vi "Configure Setpoints Limits.vi"(7 "Unit Address (1)":u8=1, 8 "error in (no error)":errorcluster, 9 "Setpoint Limit Value (0)":i16, 10 "Limit Type (False)":bool, 11 "VISA resource name":refnum<visa-resource-name>) -> (0 "error out":errorcluster, 3 "VISA resource name out":refnum<visa-resource-name>)   [LabVIEW 2014, in "Eurotherm 35xx Series.lvlib"]
doc: "This VI sets Setpoints limits."
uses:
  <instrlib>/Eurotherm 35xx Series/Eurotherm 35xx Series.lvlib
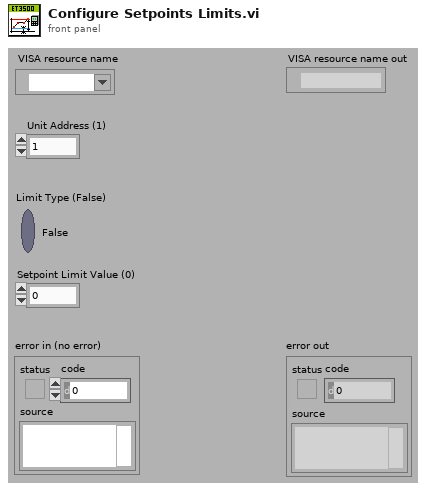
[diagram p1: front panel]
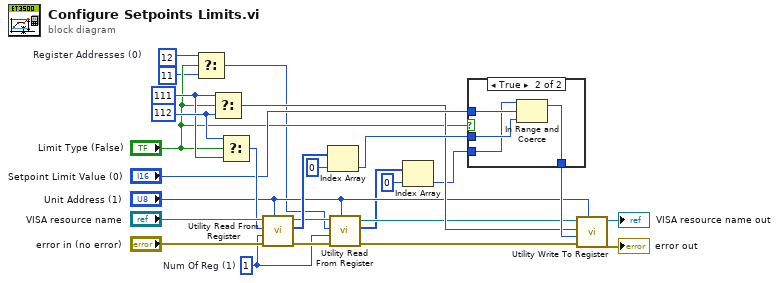
[diagram p0: block diagram]
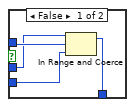
[diagram p2: hidden frame]
diagram:
  w2 = u16 1  # Num Of Reg (1)
  w22 = 112 ("Register Addresses (0)")
  w21 = 111  # Register Addresses (0)
  n1 = Select(t=12 ("Register Addresses (0)"), s="Limit Type (False)", f=11 ("Register Addresses (0)")) -> (s? t:f=w3:i32)
  n2 = Select(t=w21, s="Limit Type (False)", f=w22) -> (s? t:f=w14:i32)
  n3 = Select(t=w22, s="Limit Type (False)", f=w21) -> (s? t:f=w20:i32)
  n4 = call <instrlib>:"Utility Read From Register.vi"("Unit Address (1)"="Unit Address (1)", "error in (no error)"="error in (no error)", "Num Of Reg (1)"=w2, "Register Address (0)"=w20, "VISA resource name"="VISA resource name") -> ("error out"=w13:errorcluster, "Data"=w19:i16[], "VISA resource name out"=w10:refnum<visa-resource-name>)  [unwired: 4 in]
  n5 = Index Array(array=w19, index=0) -> (element=w17:i16)
  n6 = call <instrlib>:"Utility Read From Register.vi"("Unit Address (1)"="Unit Address (1)", "error in (no error)"=w13, "Num Of Reg (1)"=w2, "Register Address (0)"=w3, "VISA resource name"=w10) -> ("error out"=w12:errorcluster, "Data"=w7:i16[], "VISA resource name out"=w11:refnum<visa-resource-name>)  [unwired: 4 in]
  n7 = Index Array(array=w7, index=0) -> (element=w1:i16)
  n8 = case shown="True" "Limit Type (False)" {
    tunnel: w17 -> [w29 w34]
    tunnel: "Setpoint Limit Value (0)" -> [w30 w33]
    tunnel: [w28 w32] -> w15
    tunnel: w1 -> [w27 w31]
    frame False {
      n9 = In Range and Coerce(upper limit=w29, x=w30, lower limit=w27) -> (coerced(x)=w28:i16)  [unwired: 1 out]
    }
    frame True {
      n10 = In Range and Coerce(upper limit=w31, x=w33, lower limit=w34) -> (coerced(x)=w32:i16)  [unwired: 1 out]
    }
  }
  n11 = call <instrlib>:"Utility Write To Register.vi"("Unit Address (1)"="Unit Address (1)", "error in (no error)"=w12, "Data (0)"=w15, "Register Address (0)"=w14, "VISA resource name"=w11) -> ("error out"=→"error out":errorcluster, "VISA resource name out"=→"VISA resource name out":refnum<visa-resource-name>)  [unwired: 5 in]
